vi "Write Start Server.vi"(8 "error in (no error)":errorcluster, 10 "Start Server":refnum<vi>, 11 "Server UI in":refnum<class "Server UI.lvclass">) -> (0 "error out":errorcluster, 3 "Server UI out":refnum<class "Server UI.lvclass">)   [LabVIEW 2016, in "Server UI.lvlib" / "Server UI.lvclass"]
uses:
  Server UI.lvclass
  Server UI.lvclass/Server UI.ctl
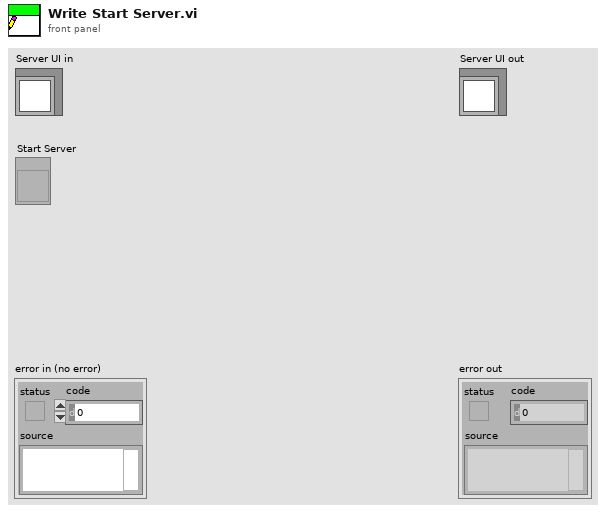
[diagram p1: front panel]
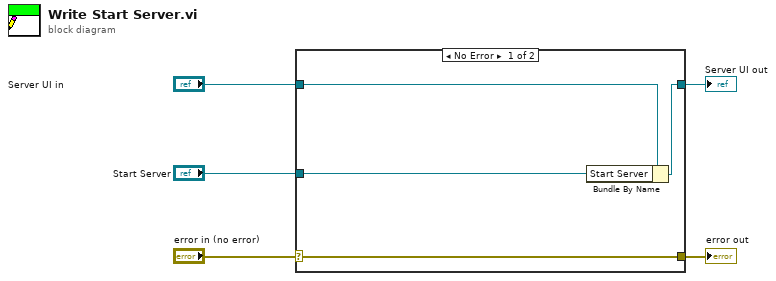
[diagram p0: block diagram]
diagram:
  n1 = case shown="No Error" "error in (no error)" {
    selector: "error in (no error)" -> [w9 w10]
    tunnel: [w9 w10] -> w4
    tunnel: [w7 w11] -> w2
    tunnel: "Server UI in" -> [w8 w11]
    tunnel: "Start Server" -> [w6 _]
    frame No Error {
      n2 = Bundle By Name(cluster=w8, "Start Server"=w6) -> (w7:refnum<class "Server UI.lvclass">)
    }
    frame Error {
    }
  }
  "error out" <- w4
  "Server UI out" <- w2
